vi "Calculate Cycle Time.vi"(11 "Coordinates":T1[](array[typedef]) {"ROI group ID" format="%#_6f"; "Laser Power (%)" format="%#_6f"; "Zoom" format="%#_6f"; "Frame Size" format="%#_6f"; "Number of lines" format="%#_6f"; "Composite ID" format="%#_6f"; "Angle (deg)" format="%#_6f"; "ROI Time (ns)" format="%#_6f"; "ROI ID" format="%#_6f"; "Pixels in ROI" format="%#_6f"; "ROI index" format="%#_6f"; "Z stop" format="%#_6f"; "Y stop" format="%#_6f"; "X stop" format="%#_6f"; "Z start" format="%#_6f"; "X start" format="%#_6f"; "Y start" format="%#_6f"}) -> (1 "AOD fill time (us)":dbl=24.16, 2 "Cycle time (us)":dbl)   [LabVIEW 2013]
uses:
  Visualisation/Functional Imaging Viewer/Typedefs/ROI parameters data type.ctl
  Typedefs/ROI ID Enum.ctl
  Global Variables/General Globals.vi
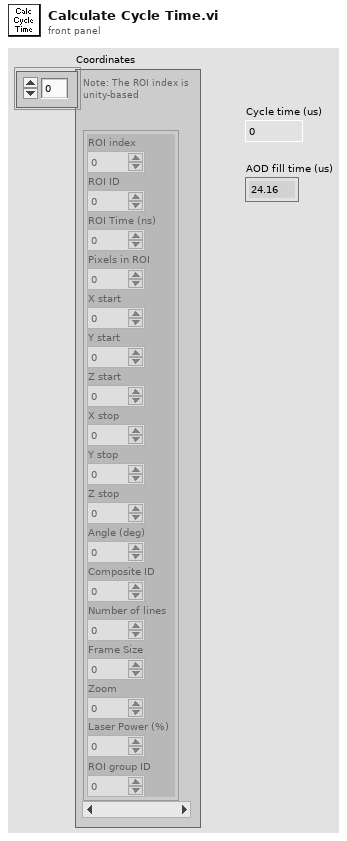
[diagram p1: front panel]
types:
  T1 = typedef "ROI parameters data type.ctl" = cluster{"ROI index":dbl, "ROI ID":dbl, "ROI Time (ns)":dbl, "Pixels in ROI":dbl, "X start":dbl, "Y start":dbl, "Z start":dbl, "X stop":dbl, "Y stop":dbl, "Z stop":dbl, "Angle (deg)":dbl, "Composite ID":dbl, "Number of lines":dbl, "Frame Size":dbl, "Zoom":dbl, "Laser Power (%)":dbl, "ROI group ID":dbl}
  T2 = typedef "ROI ID Enum.ctl" = enum16{"Point", "MiniScan", "Comp. MiniScan", "Rectangle", "Comp. volume", "Arb. plane point"}
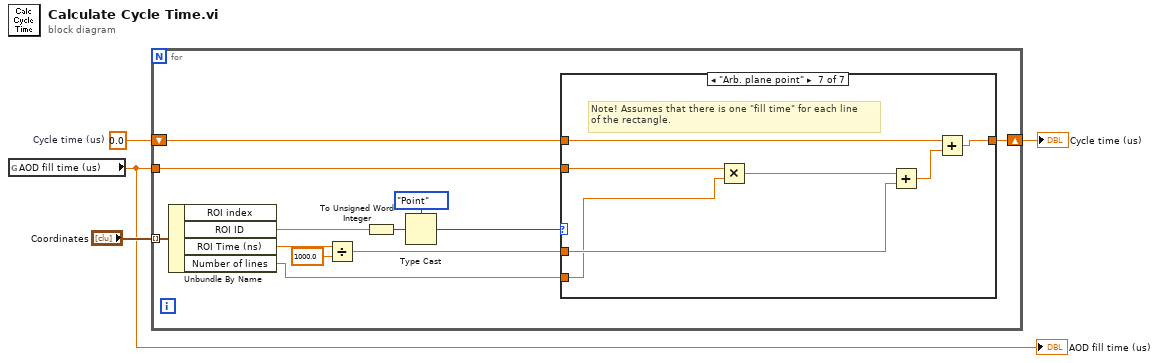
[diagram p0: block diagram]
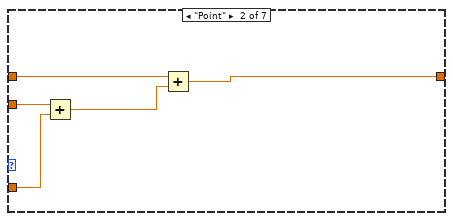
[diagram p3: hidden frame]
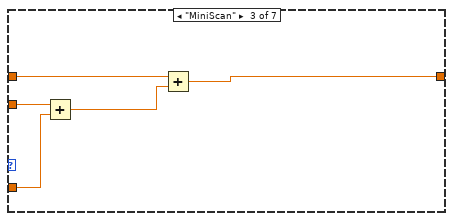
[diagram p4: hidden frame]
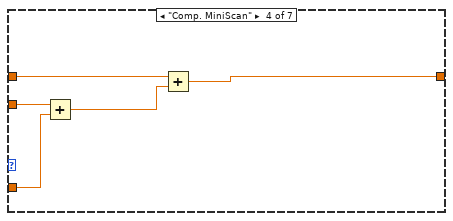
[diagram p5: hidden frame]
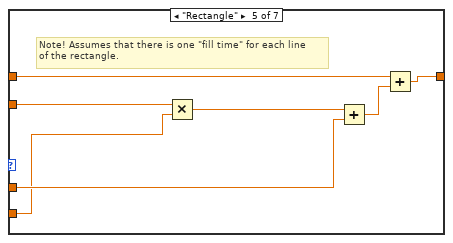
[diagram p6: hidden frame]
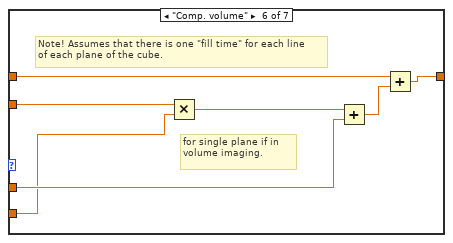
[diagram p7: hidden frame]
diagram:
  w3 = 0.0  # Cycle time (us)
  n1 = global read "General Globals.vi" "AOD fill time (us)"() -> (w2:dbl)
  "AOD fill time (us)" <- w2
  n2 = for {
    tunnel: "Coordinates" -> [w16] mode=indexing
    tunnel: w2 -> [w15]
    shift-right: [w14] -> w1
    shift-left: w3 -> [w13]
    n3 = Unbundle By Name(w16) -> ("ROI ID"=w12:dbl, "ROI Time (ns)"=w7:dbl, "Number of lines"=w5:dbl)  [unwired: 1 out]
    n4 = Divide(x=w7, y=1000.0) -> (x/y=w6:dbl)
    n5 = To Unsigned Word Integer(number=w12) -> (unsigned 16bit integer=w10:u16)
    n6 = Type Cast(type=ROI_ID_Enum."Point" ("ROI ID Enum"), x=w10) -> (*(type *) &x=w9:T2)
    n7 = case shown="\"Arb. plane point\"" w9 {
      tunnel: w6 -> [_ w22 w27 w32 w39 w46 w53]
      tunnel: w15 -> [_ w21 w26 w31 w35 w42 w49]
      tunnel: [w17 w20 w25 w30 w38 w45 w52] -> w14
      tunnel: w13 -> [w17 w19 w24 w29 w37 w44 w51]
      tunnel: w5 -> [_ _ _ _ w33 w41 w47]
      frame Default {
      }
      frame "Point" {
        n8 = Add(x=w21, y=w22) -> (x+y=w18:dbl)
        n9 = Add(x=w19, y=w18) -> (x+y=w20:dbl)
      }
      frame "MiniScan" {
        n10 = Add(x=w26, y=w27) -> (x+y=w23:dbl)
        n11 = Add(x=w24, y=w23) -> (x+y=w25:dbl)
      }
      frame "Comp. MiniScan" {
        n12 = Add(x=w31, y=w32) -> (x+y=w28:dbl)
        n13 = Add(x=w29, y=w28) -> (x+y=w30:dbl)
      }
      frame "Rectangle" {
        # "Note! Assumes that there is one \"fill time\" for each line\nof the rectangle."
        n14 = Multiply(x=w35, y=w33) -> (x*y=w34:dbl)
        n15 = Add(x=w34, y=w39) -> (x+y=w36:dbl)
        n16 = Add(x=w37, y=w36) -> (x+y=w38:dbl)
      }
      frame "Comp. volume" {
        # "for single plane if in volume imaging."
        # "Note! Assumes that there is one \"fill time\" for each line\nof each plane of the cube."
        n17 = Multiply(x=w42, y=w41) -> (x*y=w40:dbl)
        n18 = Add(x=w40, y=w46) -> (x+y=w43:dbl)
        n19 = Add(x=w44, y=w43) -> (x+y=w45:dbl)
      }
      frame "Arb. plane point" {
        # "Note! Assumes that there is one \"fill time\" for each line\nof the rectangle."
        n20 = Multiply(x=w49, y=w47) -> (x*y=w48:dbl)
        n21 = Add(x=w48, y=w53) -> (x+y=w50:dbl)
        n22 = Add(x=w51, y=w50) -> (x+y=w52:dbl)
      }
    }
  }
  "Cycle time (us)" <- w1
